vi "create_data_header_units_heat_measurement.vi"() -> (2 "header units":string)   [LabVIEW 2019]
uses:
  Global Variables/global.vi
  Instrument_Setup.vi
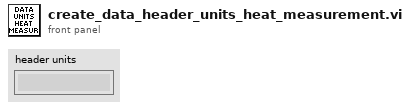
[diagram p1: front panel]
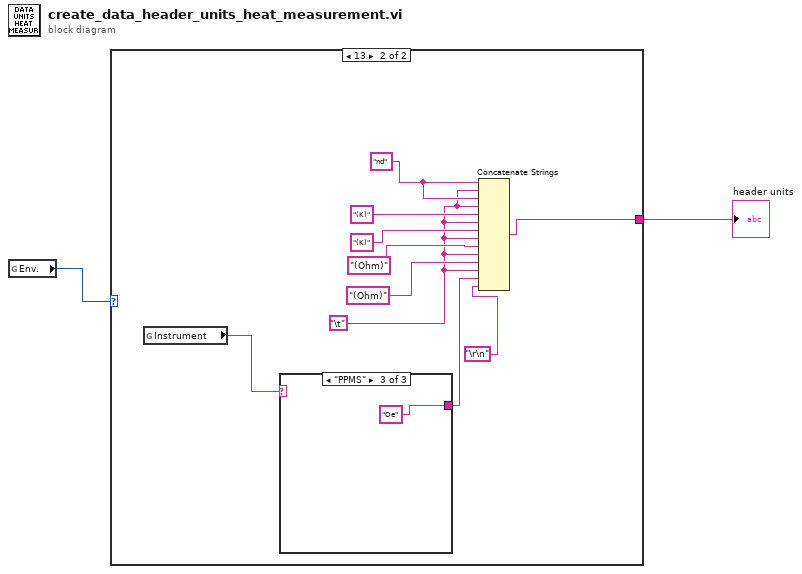
[diagram p0: block diagram]
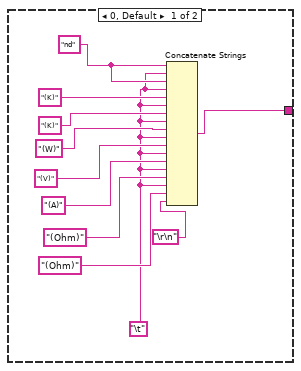
[diagram p2: hidden frame]
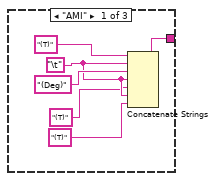
[diagram p3: hidden frame]
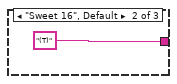
[diagram p4: hidden frame]
diagram:
  n1 = global read "global.vi" "Env."() -> (w1:i32)
  n2 = case shown="13" w1 {
    tunnel: [w5 w18] -> w2
    frame 0, Default {
      w3 = "\t"
      w4 = "nd"
      n3 = Concatenate Strings(w4, w3, w4, w3, "(K)", w3, "(K)", w3, "(W)", w3, "(V)", w3, "(A)", w3, "(Ohm)", w3, "(Ohm)", "\r\n") -> (w5:string)
    }
    frame 13 {
      w17 = "\t"
      w19 = "nd"
      n4 = global read "Instrument_Setup.vi" "Instrument"() -> (w15:string)
      n5 = case shown="\"PPMS\"" w15 {
        tunnel: [w27 "(T)" "Oe"] -> w14
        frame "AMI" {
          w26 = "\t"
          n6 = Concatenate Strings("(T)", w26, "(Deg)", w26, "(T)", w26, "(T)") -> (w27:string)
        }
        frame "Sweet 16", Default {
        }
        frame "PPMS" {
        }
      }
      n7 = Concatenate Strings(w19, w17, w19, w17, "(K)", w17, "(K)", w17, "(Ohm)", w17, "(Ohm)", w17, w14, "\r\n") -> (w18:string)
    }
  }
  "header units" <- w2
